vi "MC-BonOMM_talker.vi"(0 "MC-BonOMM VRN":refnum<visa-resource-name>="COM3", 1 "Commande":string, 2 "byte count":u32=1, 3 "Timeout (ms)":i32, 4 "answer=command?":bool=TRUE) -> (5 "Answer":string, 6 "ok ?":bool)   [LabVIEW 2019]
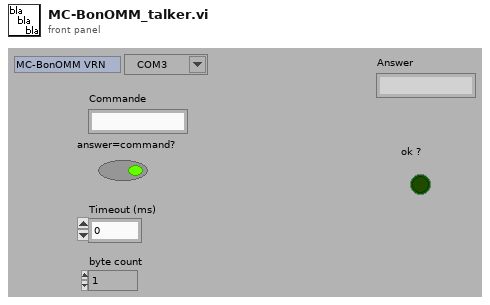
[diagram p1: front panel]
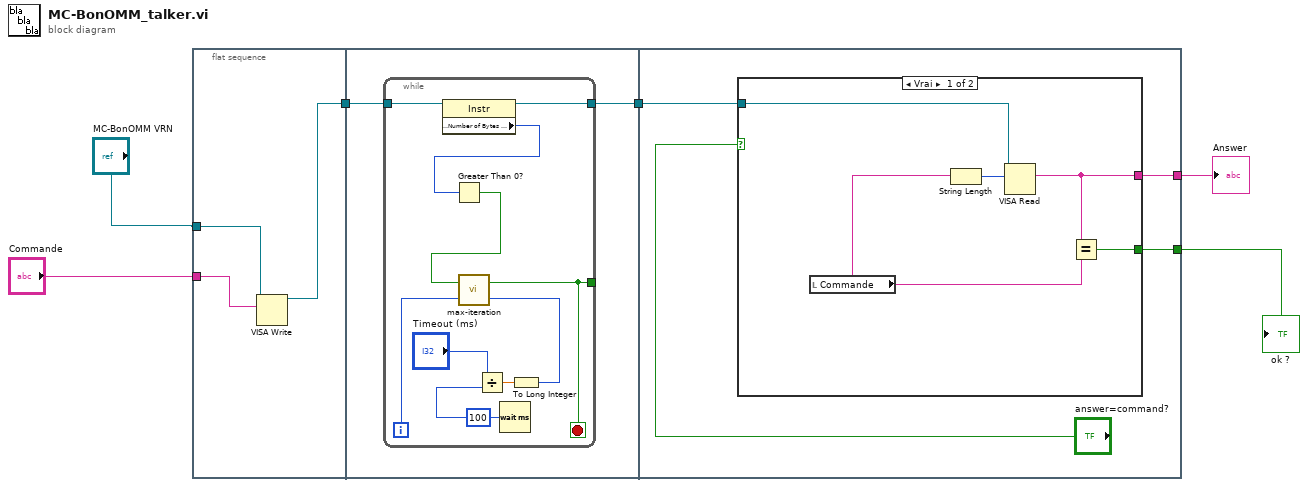
[diagram p0: block diagram]
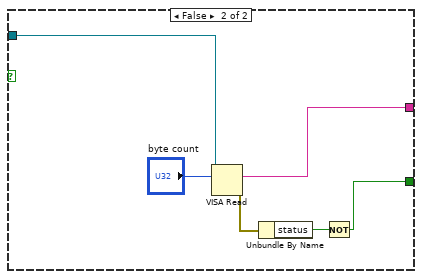
[diagram p2: hidden frame]
diagram:
  n1 = flat-sequence {
    tunnel: "MC-BonOMM VRN" -> [w9]
    tunnel: "Commande" -> [w8]
    tunnel: [w7] -> w4
    tunnel: w4 -> [w11]
    tunnel: [w10] -> w3
    tunnel: w3 -> [w24]
    tunnel: [w23] -> w2
    tunnel: [w22] -> w1
    frame #0 {
      n2 = VISA Write(VISA resource name=w9, write buffer=w8) -> (VISA resource name out=w7:refnum<visa-resource-name>)  [unwired: 1 in, 2 out]
    }
    frame #1 {
      n3 = while {
        tunnel: w11 -> [w21]
        tunnel: [w20] -> w10
        tunnel: [w16] -> _
        i -> [w17]
        stop <- w16 stop-if-true
        w14 = u32 100 ("milliseconds to wait")
        n4 = property class="Instr"(reference=w21) -> (reference out=w20:refnum<visa-resource-name>, "Serial Settings:Number of Bytes at Serial Port"=w19:u32)  [unwired: 1 in, 1 out]
        n5 = Greater Than 0?(x=w19) -> (x > 0?=w18:bool)
        n6 = Divide(x="Timeout (ms)", y=w14) -> (x/y=w13:dbl)
        n7 = Wait (ms)(milliseconds to wait=w14) -> ()  [unwired: 1 out]
        n8 = To Long Integer(number=w13) -> (32bit integer=w12:i32)
        n9 = call "max-iteration.vi"("i max"=w12, "i act"=w17, "Valeur entrante"=w18) -> ("break ?"=w16:bool)
      }
    }
    frame #2 {
      n10 = case shown="Vrai" "answer=command?" {
        tunnel: w24 -> [w30 w36]
        tunnel: [w29 w31] -> w23
        tunnel: [w26 w32] -> w22
        frame True {
          n11 = local read "Commande"() -> (w27:string)
          n12 = String Length(string=w27) -> (length=w28:i32)
          n13 = VISA Read(VISA resource name=w30, byte count=w28) -> (read buffer=w26:string)  [unwired: 1 in, 3 out]
          n14 = Equal?(x=w26, y=w27) -> (x = y?=w29:bool)
        }
        frame False {
          n15 = VISA Read(VISA resource name=w36, byte count="byte count") -> (read buffer=w32:string, error out=w34:errorcluster)  [unwired: 1 in, 2 out]
          n16 = Unbundle By Name(w34) -> ("status"=w33:bool)
          n17 = Not(x=w33) -> (.not. x?=w31:bool)
        }
      }
    }
  }
  "ok ?" <- w2
  "Answer" <- w1
